vi "AddTestMethod_Provider_OnPopupMenu.vi"(11 "objects":T1[](array[typedef])) -> ()   [LabVIEW 2013]
uses:
  <resource>/Framework/Providers/API/ItemRef.ctl
  <resource>/Framework/Providers/API/mxLvMenuItem.ctl
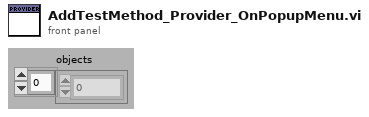
[diagram p1: front panel]
types:
  T1 = typedef "ItemRef.ctl" = u64
  T2 = typedef "mxLvMenuItem.ctl" = cluster{"Menu Name":string, "Description":string, "Icon File Name":path, "Menu Tag":string, "Enabled":bool, "Checked":bool, "Separator":bool, "Batchable":bool, "Weight":i32, "Batch Mode (Ignored if Not Batchable)":enum32{"Show If All Items Support Command", "Show If Any Items Support Command"}, "Menu Location":enum32{"<None>", "Project", "Project / Build Specifications", "Tools", "Tools / Source Control", "Tools / Real-Time Module", "Help"}, "Exclude From Getting Started Window Menu":bool}
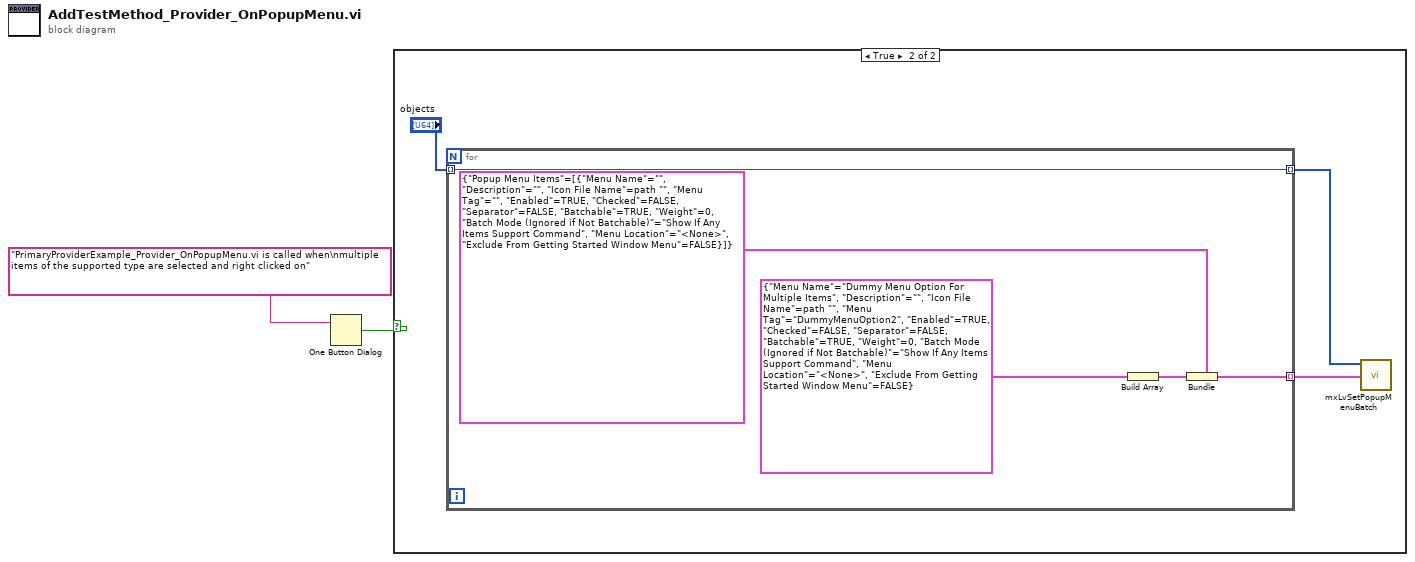
[diagram p0: block diagram]
diagram:
  n1 = One Button Dialog(message="PrimaryProviderExample_Provider_OnPopupMenu.vi is called when\nmultiple items of the supported type are selected and right clicked on") -> (true=w2:bool)  [unwired: 1 in]
  n2 = case shown="True" w2 {
    frame False {
    }
    frame True {
      n3 = for {
        tunnel: [w8] -> w5 mode=indexing
        tunnel: "objects" -> [w6] mode=indexing
        tunnel: [w6] -> w3 mode=indexing
        n4 = Build Array(T2 {"Menu Name"="Dummy Menu Option For Multiple Items", "Description"="", "Icon File Name"=path "", "Menu Tag"="DummyMenuOption2", "Enabled"=TRUE, "Checked"=FALSE, "Separator"=FALSE, "Batchable"=TRUE, "Weight"=0, "Batch Mode (Ignored if Not Batchable)"=enum."Show If Any Items Support Command", "Menu Location"=enum."<None>", "Exclude From Getting Started Window Menu"=FALSE} ("Menu Item")) -> (w9:T2[])
        n5 = Bundle(cluster=cluster{"Popup Menu Items":T2[]} {"Popup Menu Items"=[{"Menu Name"="", "Description"="", "Icon File Name"=path "", "Menu Tag"="", "Enabled"=TRUE, "Checked"=FALSE, "Separator"=FALSE, "Batchable"=TRUE, "Weight"=0, "Batch Mode (Ignored if Not Batchable)"=enum."Show If Any Items Support Command", "Menu Location"=enum."<None>", "Exclude From Getting Started Window Menu"=FALSE}]}, "Popup Menu Items"=w9) -> (w8:cluster{"Popup Menu Items":T2[]})
      }
      n6 = call <resource>:"mxLvSetPopupMenuBatch.vi"("Menu Items"=w5, "Items"=w3) -> ()  [unwired: 8 in, 2 out]
    }
  }
